vi "Práctica 2_Dídier Javier Ramírez Henao.vi"() -> ()   [LabVIEW 2020]
panel:
  out "Banda":bool
  out "Ventilador":bool
  in  "Parar":bool
  in  "Inicio":bool
  out "Motor":bool
  out "Horno":bool
  # "Dídier Javier Ramírez Henao"
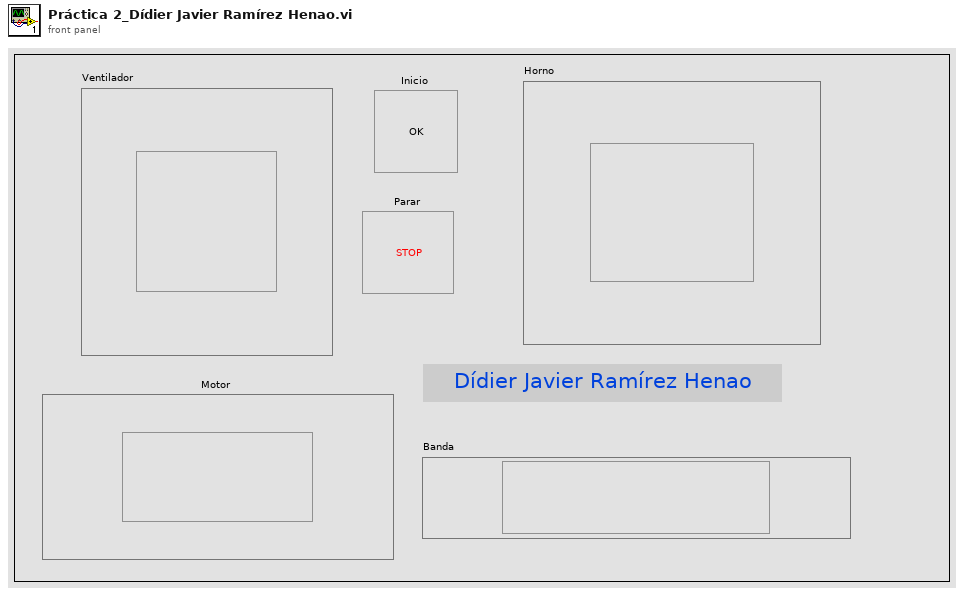
[diagram p1: front panel]
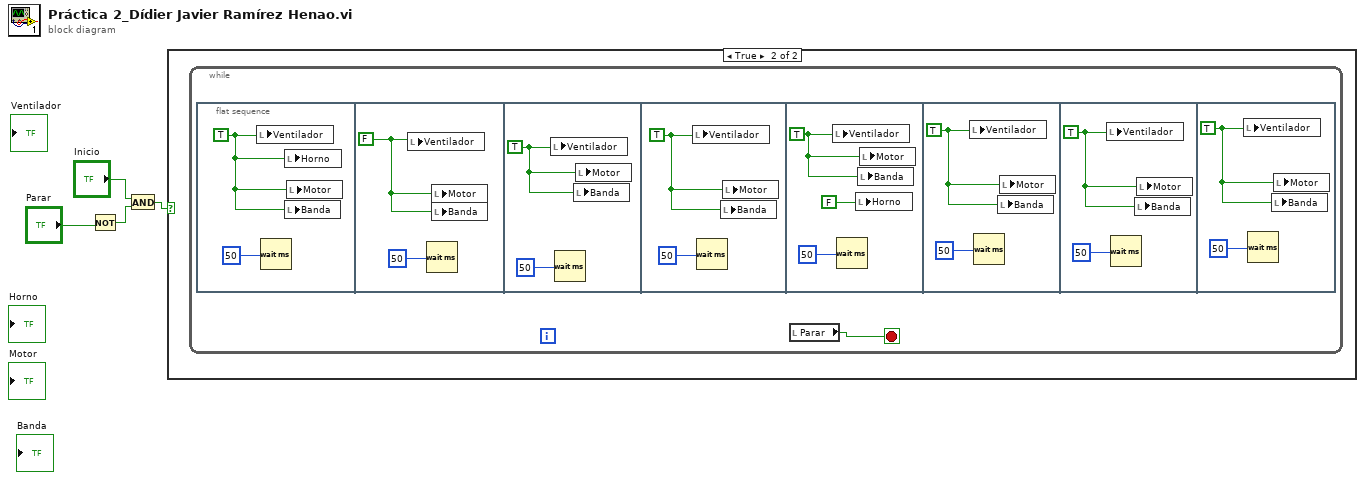
[diagram p0: block diagram]
diagram:
  n1 = Not(x="Parar") -> (.not. x?=w2:bool)
  n2 = And(x="Inicio", y=w2) -> (x .and. y?=w4:bool)
  n3 = case shown="True" w4 {
    frame False {
    }
    frame True {
      n4 = while {
        stop <- w5 stop-if-true
        n5 = flat-sequence {
          frame #0 {
            w6 = TRUE
            n6 = local write "Ventilador"(w6) -> ()
            n7 = Wait (ms)(milliseconds to wait=50) -> ()  [unwired: 1 out]
            n8 = local write "Horno"(w6) -> ()
            n9 = local write "Banda"(w6) -> ()
            n10 = local write "Motor"(w6) -> ()
          }
          frame #1 {
            w8 = FALSE
            n11 = local write "Ventilador"(w8) -> ()
            n12 = Wait (ms)(milliseconds to wait=50) -> ()  [unwired: 1 out]
            n13 = local write "Motor"(w8) -> ()
            n14 = local write "Banda"(w8) -> ()
          }
          frame #2 {
            w11 = TRUE
            n15 = local write "Ventilador"(w11) -> ()
            n16 = Wait (ms)(milliseconds to wait=50) -> ()  [unwired: 1 out]
            n17 = local write "Banda"(w11) -> ()
            n18 = local write "Motor"(w11) -> ()
          }
          frame #3 {
            w12 = TRUE
            n19 = local write "Ventilador"(w12) -> ()
            n20 = Wait (ms)(milliseconds to wait=50) -> ()  [unwired: 1 out]
            n21 = local write "Banda"(w12) -> ()
            n22 = local write "Motor"(w12) -> ()
          }
          frame #4 {
            w16 = TRUE
            n23 = local write "Ventilador"(w16) -> ()
            n24 = Wait (ms)(milliseconds to wait=50) -> ()  [unwired: 1 out]
            n25 = local write "Horno"(FALSE) -> ()
            n26 = local write "Banda"(w16) -> ()
            n27 = local write "Motor"(w16) -> ()
          }
          frame #5 {
            w17 = TRUE
            n28 = local write "Ventilador"(w17) -> ()
            n29 = Wait (ms)(milliseconds to wait=50) -> ()  [unwired: 1 out]
            n30 = local write "Banda"(w17) -> ()
            n31 = local write "Motor"(w17) -> ()
          }
          frame #6 {
            w20 = TRUE
            n32 = local write "Ventilador"(w20) -> ()
            n33 = Wait (ms)(milliseconds to wait=50) -> ()  [unwired: 1 out]
            n34 = local write "Banda"(w20) -> ()
            n35 = local write "Motor"(w20) -> ()
          }
          frame #7 {
            w21 = TRUE
            n36 = local write "Ventilador"(w21) -> ()
            n37 = Wait (ms)(milliseconds to wait=50) -> ()  [unwired: 1 out]
            n38 = local write "Banda"(w21) -> ()
            n39 = local write "Motor"(w21) -> ()
          }
        }
        n40 = local read "Parar"() -> (w5:bool)
      }
    }
  }
